vi "SNStrComp.vi"(10 "POWER Board S/N":string, 11 "DSP Board S/N":string) -> (2 "Boolean":bool=TRUE)   [LabVIEW 2017]
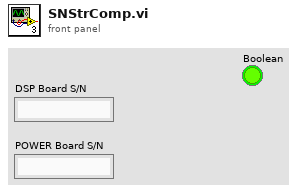
[diagram p1: front panel]
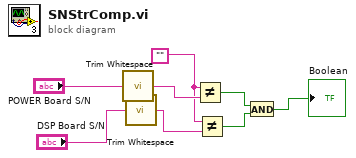
[diagram p0: block diagram]
diagram:
  w5 = ""
  n1 = call <vilib>:"Trim Whitespace.vi"("string"="POWER Board S/N") -> ("trimmed string"=w6:string)  [unwired: 1 in]
  n2 = call <vilib>:"Trim Whitespace.vi"("string"="DSP Board S/N") -> ("trimmed string"=w4:string)  [unwired: 1 in]
  n3 = Not Equal?(x=w5, y=w6) -> (x != y?=w2:bool)
  n4 = Not Equal?(x=w5, y=w4) -> (x != y?=w3:bool)
  n5 = And(x=w2, y=w3) -> (x .and. y?=→"Boolean":bool)
